vi "CoordRunAll.vi"(0 "Refnum in":T3, 1 "CoordinatteEntry In":T4 {"AnalysisSetting"."OriginPointInfo"."Mode" items=["Horizontal Motion", "Vertical Motion", "Horizontal and Vertical Motion", "Horizontal. Vertical and Angular Motion"]; "AnalysisSetting"."ROI"."Contours"."Type" items=["No Selection", "Point", "Line", "Rectangle", "Oval", "Polygon", "Freehand Region", "Annulus", "Unused2", "Unused3", "Broken Line", "Freehand Line", "Rotated Rectangle"]}, 4 "AnalysisSetting":T1[](array[typedef]) {"OriginPointInfo"."Mode" items=["Horizontal Motion", "Vertical Motion", "Horizontal and Vertical Motion", "Horizontal. Vertical and Angular Motion"]; "ROI"."Contours"."Type" items=["No Selection", "Point", "Line", "Rectangle", "Oval", "Polygon", "Freehand Region", "Annulus", "Unused2", "Unused3", "Broken Line", "Freehand Line", "Rotated Rectangle"]}, 5 "Error In":errorcluster, 7 "CoordSystemRun?":bool, 9 "CreatDllImage":bool, 11 "RootPath":path, 13 "Dllindex":i32) -> (15 "CoordinatteEntry Out":T4 {"AnalysisSetting"."OriginPointInfo"."Mode" items=["Horizontal Motion", "Vertical Motion", "Horizontal and Vertical Motion", "Horizontal. Vertical and Angular Motion"]; "AnalysisSetting"."ROI"."Contours"."Type" items=["No Selection", "Point", "Line", "Rectangle", "Oval", "Polygon", "Freehand Region", "Annulus", "Unused2", "Unused3", "Broken Line", "Freehand Line", "Rotated Rectangle"]}, 18 "Main Out":T7[](array[typedef]), 19 "Error Out":errorcluster)   [LabVIEW 2015]
uses:
  Controls/Vision_DataEntry.ctl
  Process/Controls/Process_Setting.ctl
  Process/Controls/Process_Type.ctl
  Analysis/Controls/Analysis_Setting.ctl
  Analysis/Controls/Analysis_Type.ctl
  Control/CoordinatteEntry.ctl
  Control/CoordinateAnalysisSetting.ctl
  <vilib>/vision/Image Controls.llb/IMAQ Image.ctl
  Control/DataTransform.ctl
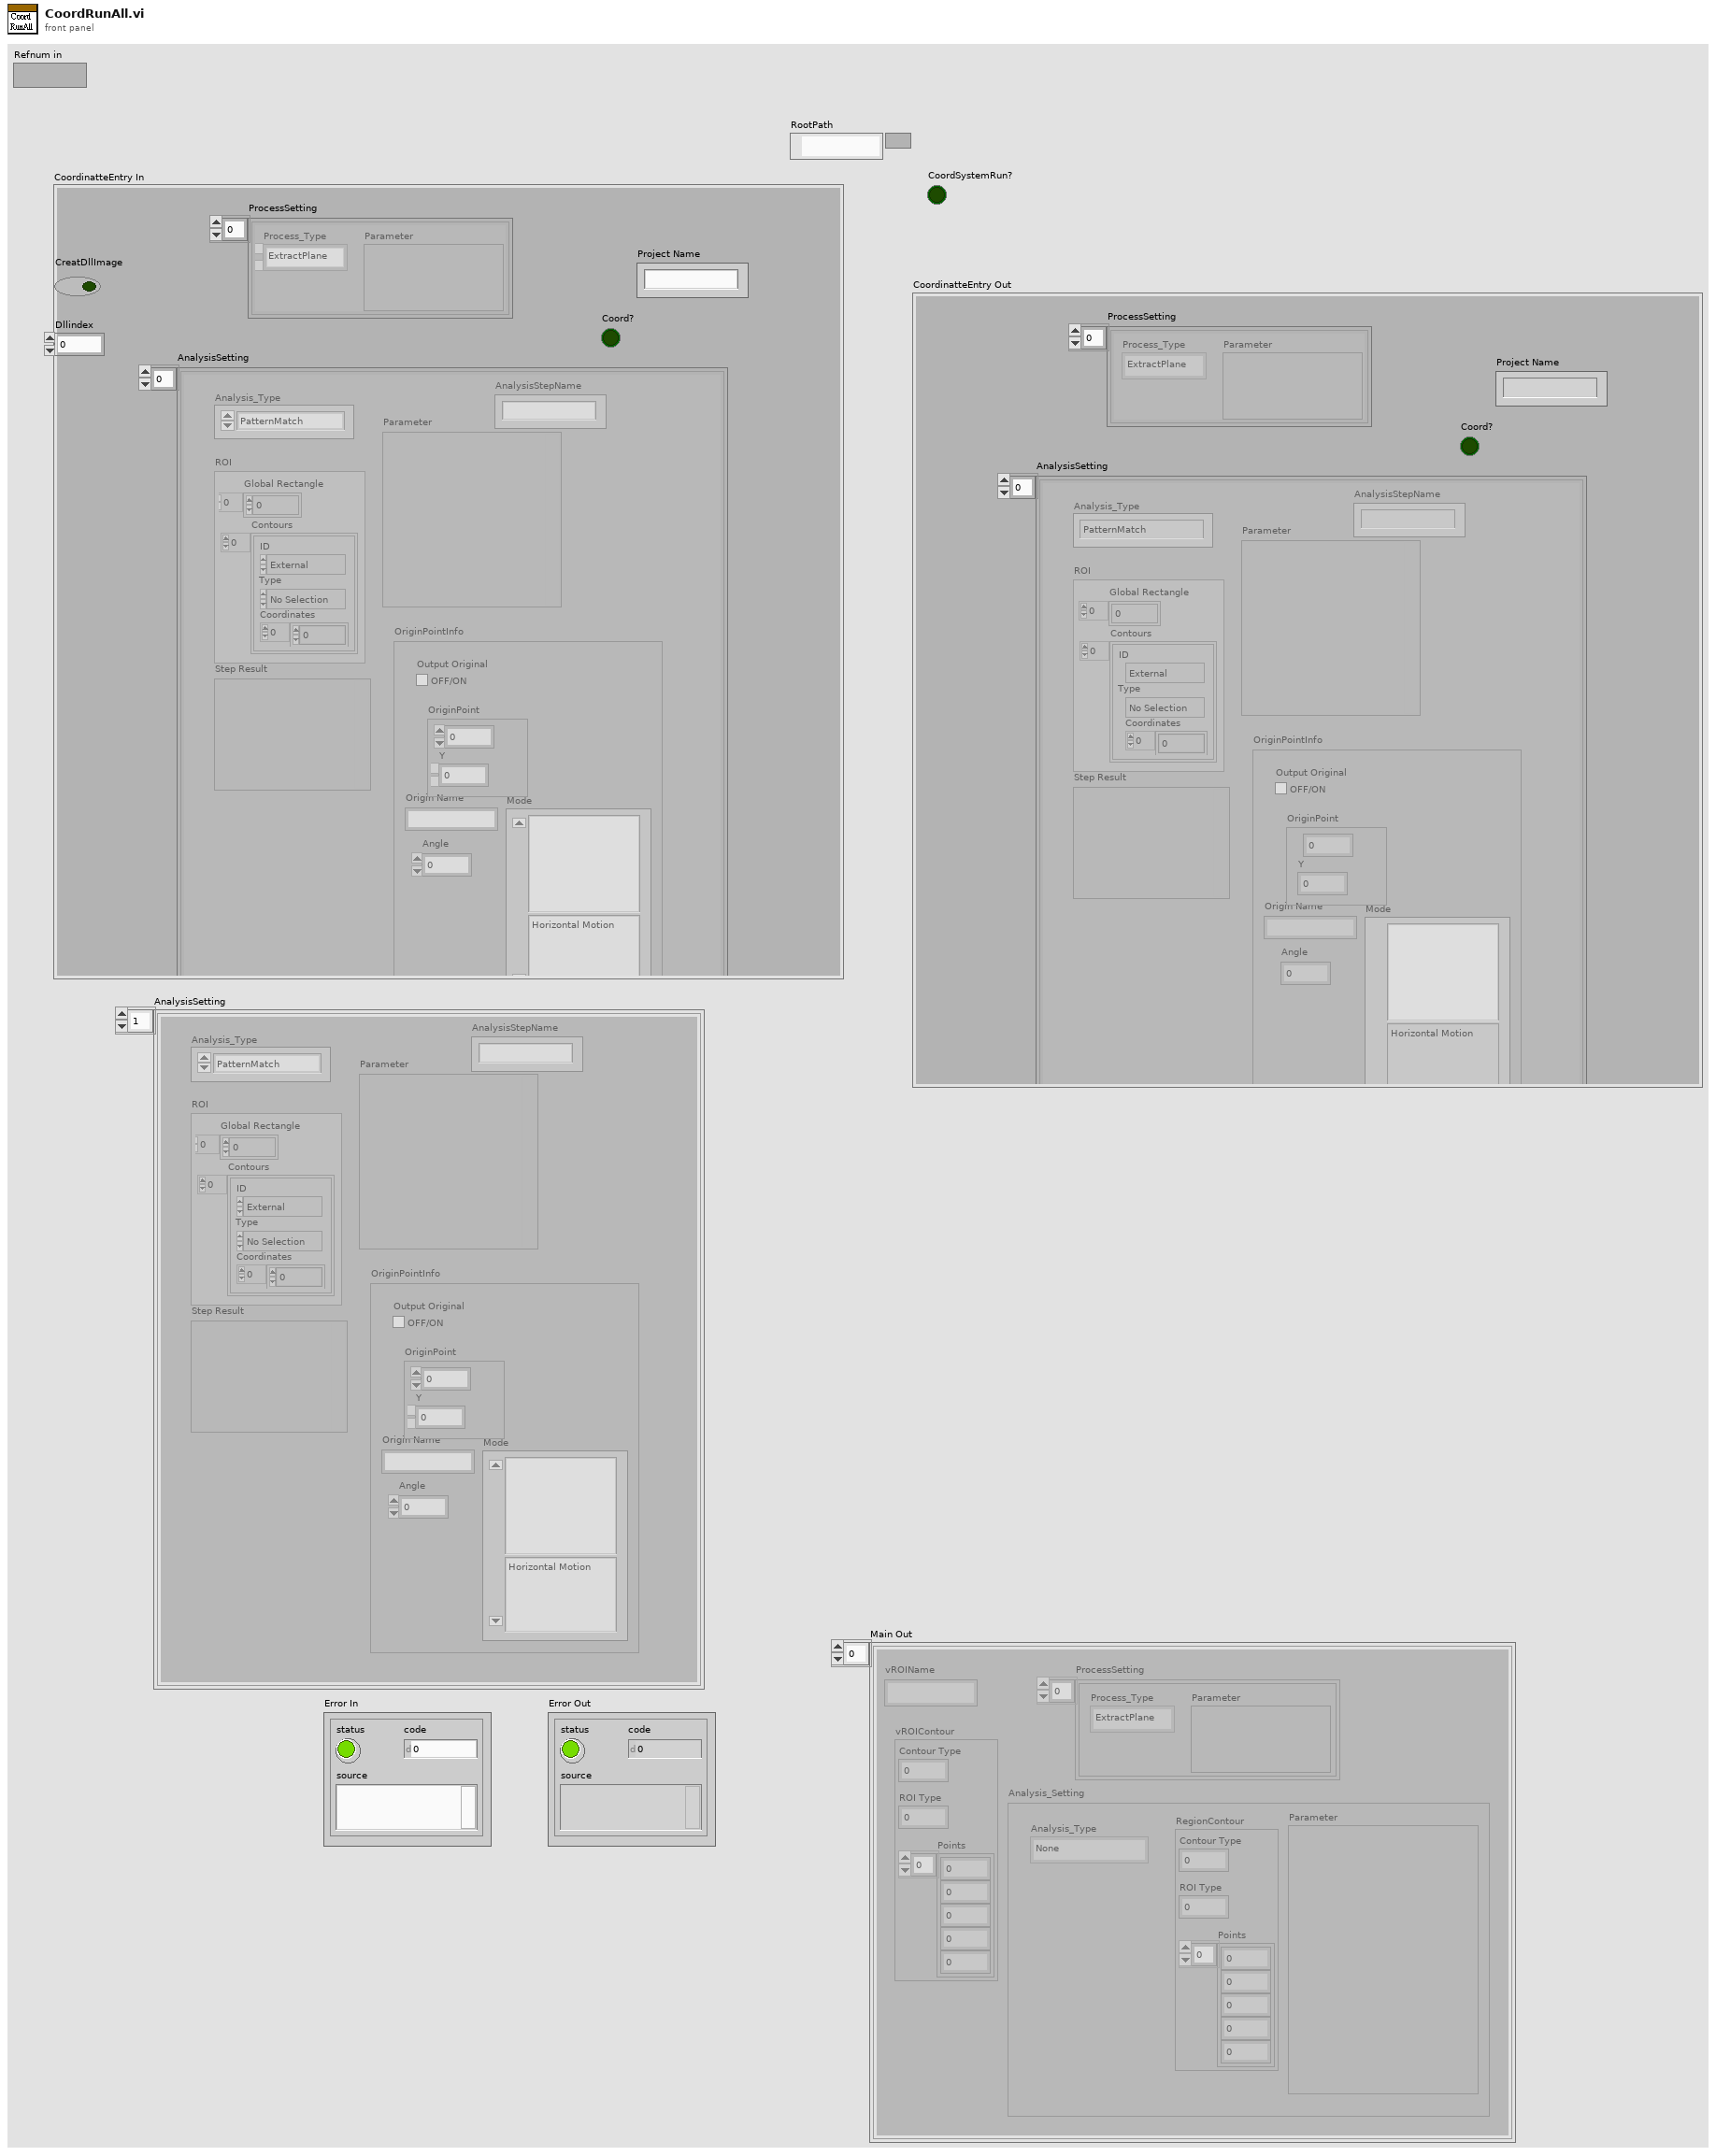
[diagram p1: front panel]
types:
  T1 = typedef "CoordinateAnalysisSetting.ctl" = cluster{"Analysis_Type":enum16{"PatternMatch", "Straight Edge"}, "ROI ":T2, "Parameter":variant, "Step Result":variant, "OriginPointInfo":cluster{"Output Original":bool, "Origin Name":string, "Angle":dbl, "Mode":u16, "OriginPoint":cluster{"X":dbl, "Y":dbl}}, "AnalysisStepName":string}
  T2 = typedef "ROI Descriptor" = cluster{"Global Rectangle":i32[], "Contours":cluster{"ID":enum32{"External", "Internal"}, "Type":u32, "Coordinates":i32[]}[]}
  T3 = typedef "IMAQ Image.ctl" = refnum<image>
  T4 = typedef "CoordinatteEntry.ctl" = cluster{"ProcessSetting":T5[], "Project Name":string, "AnalysisSetting":T1[], "Coord?":bool}
  T5 = typedef "Process_Setting.ctl" = cluster{"Process_Type":T6, "Parameter":variant}
  T6 = typedef "Process_Type.ctl" = enum16{"None", "ExtractPlane", "BinaryMono", "Operators", "GrayMorphology", "Filters", "Lookup Table", "Particle Filter"}
  T7 = typedef "Vision_DataEntry.ctl" = cluster{"vROIName":string, "vROIContour":cluster{"Contour Type":u32, "ROI Type":u32, "Points":i32[]}, "ProcessSetting":T5[], "Analysis_Setting":T8}
  T8 = typedef "Analysis_Setting.ctl" = cluster{"Analysis_Type":T9, "RegionContour":cluster{"Contour Type":u32, "ROI Type":u32, "Points":i32[]}, "Parameter":variant}
  T9 = typedef "Analysis_Type.ctl" = enum16{"None", "PatternMatch", "Edge Detection", "Barcode 1D", "Barcode 2D", "Clamp", "Clamp MAX", "Particle", "LCD", "Straight Edge"}
  T10 = typedef "DataTransform.ctl" = enum16{"CoordToMain", "MainToCoord"}
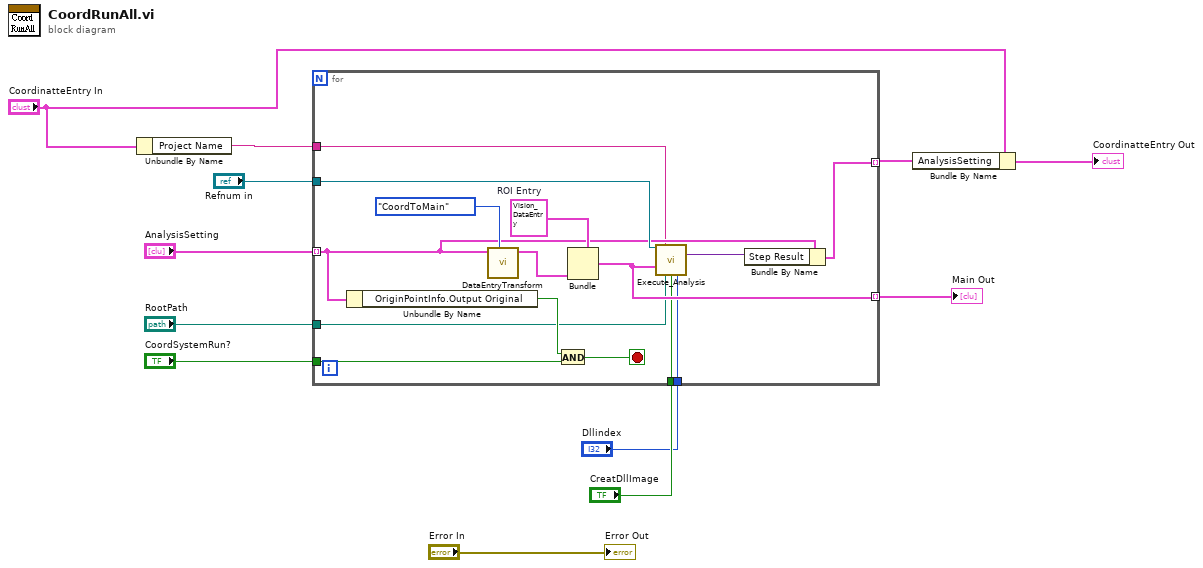
[diagram p0: block diagram]
diagram:
  n1 = Unbundle By Name("CoordinatteEntry In") -> ("Project Name"=w5:string)
  n2 = for {
    tunnel: "AnalysisSetting" -> [w20] mode=indexing
    tunnel: "Refnum in" -> [w24]
    tunnel: [w23] -> w12 mode=indexing
    tunnel: [w21] -> w11 mode=indexing
    tunnel: "CoordSystemRun?" -> [w18]
    tunnel: w5 -> [w16]
    tunnel: "RootPath" -> [w15]
    tunnel: "CreatDllImage" -> [w14]
    tunnel: "Dllindex" -> [w13]
    stop <- w17 stop-if-true
    w27 = T7 {"vROIName"="", "vROIContour"={"Contour Type"=0, "ROI Type"=0, "Points"=[]}, "ProcessSetting"=[], "Analysis_Setting"={"Analysis_Type"=enum."None", "RegionContour"={"Contour Type"=0, "ROI Type"=0, "Points"=[]}, "Parameter"=variant}}  # ROI Entry
    n3 = Unbundle By Name(w20) -> ("OriginPointInfo.Output Original"=w19:bool)
    n4 = call "DataEntryTransform.vi"("DataTrasform"=DataTransform."CoordToMain", "CoordSettingIn"=w20) -> ("MainSettingOut"=w25:T8)  [unwired: 7 in, 2 out]
    n5 = And(x=w19, y=w18) -> (x .and. y?=w17:bool)
    n6 = Bundle(cluster=w27, "Analysis_Setting"=w25) -> (w21:T7)  [unwired: 3 in]
    n7 = call "Execute_Analysis.vi"("Image In"=w24, "ProjectName"=w16, "ROI Entry"=w21, "RootPath"=w15, "CreatDllImage"=w14, "Script Index"=w13) -> ("Result"=w22:variant)  [unwired: 6 in, 3 out]
    n8 = Bundle By Name(cluster=w20, "Step Result"=w22) -> (w23:T1)
  }
  "Main Out" <- w11
  n9 = Bundle By Name(cluster="CoordinatteEntry In", "AnalysisSetting"=w12) -> (→"CoordinatteEntry Out":T4)
  "Error Out" <- "Error In"
